vi "RAMP_init_ramp_scan_FPGA.vi"(0 "queue CAMERA":refnum<queue>, 1 "queue piezo":refnum<queue>, 3 "queue DAQ":refnum<queue>, 4 "queue ASI stage":refnum<queue>, 5 "Laser lines array":dbl[][](array[numeric]), 7 "error in":errorcluster, 8 "Illumination source":bool, 9 "Brightfield intensity":dbl, 10 "Display?":bool=TRUE, 12 "Autofocus":bool, 13 "Movie path":path, 14 "Total range (nm)":u32=2000, 15 "z step (nm)":u32=50, 16 "Start acquisition":bool, 17 "Exp time (s)":sgl=0.05 format="%#_3g", 21 "queue FPGA":refnum<queue>, 25 "Measure QPD":bool) -> (20 "Ramp":dbl[](array[numeric]), 23 "Total # z steps":i32, 24 "Ready":bool, 27 "error out":errorcluster)   [LabVIEW 2015]
uses:
  CONTROLS/Q_MCL_piezo_element.ctl
  CONTROLS/Q_camera_element.ctl
  CONTROLS/Q_ASI_stage_element.ctl
  CONTROLS/Q_DAQ_element.ctl
  CONTROLS/Q_FPGA_element.ctl
  GLOBAL/Global_ASI_stage.vi
  GLOBAL/Global_MCL_piezo.vi
  GLOBAL/Global_DAQ.vi
  GLOBAL/Global_CAMERA.vi
  GLOBAL/Global_FPGA.vi
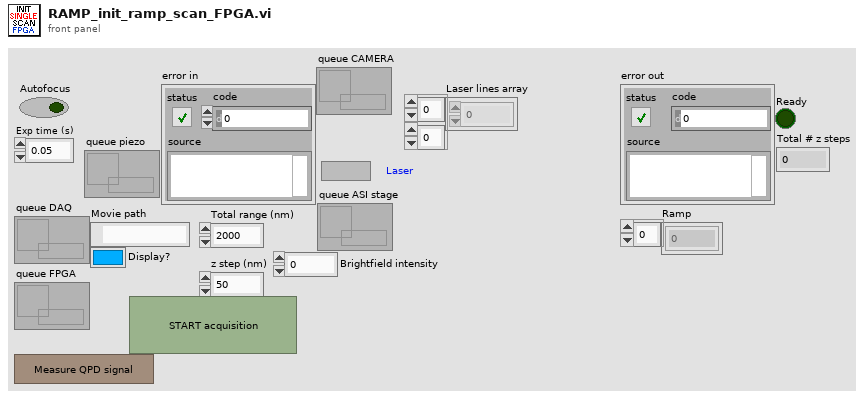
[diagram p1: front panel]
types:
  T1 = typedef "Q_DAQ_element.ctl" = cluster{"variant":variant, "Instruction":enum16{"DAQ_idle", "DAQ_initialize", "DAQ_error", "DAQ_security_stop", "DAQ_init_single_scan", "DAQ_single_scan", "DAQ_init_merFISH", "DAQ_scan_merFISH", "DAQ_photobleaching_merFISH", "DAQ_close_merFISH", "DAQ_stop"}}
  T2 = typedef "Q_camera_element.ctl" = cluster{"variant":variant, "Instruction":enum16{"CAMERA_idle", "CAMERA_initialize", "CAMERA_error", "CAMERA_security_stop", "CAMERA_not_acquiring", "CAMERA_acquiring", "CAMERA_start_acquiring", "CAMERA_stop_acquiring", "CAMERA_change_exposure", "CAMERA_define_ROI", "CAMERA_cooler", "CAMERA_acquire_movie", "CAMERA_init_scan", "CAMERA_check_image_scan", "CAMERA_close_scan", "CAMERA_init_merFISH", "CAMERA_start_acquiring_merFISH", "CAMERA_close_scan_merFISH", "CAMERA_close_merFISH", "CAMERA_STOP"}}
  T3 = cluster{"N laser lines":i32, "N Z positions":i32, "Laser lines":i32[], "Laser power":sgl[], "Measure QPD":bool}
  T4 = typedef "Q_FPGA_element.ctl" = cluster{"variant":variant, "Instruction":enum16{"FPGA_idle", "FPGA_initialize", "FPGA_error", "FPGA_security_stop", "FPGA_laser", "FPGA_start_stop_measure_QPD", "FPGA_measure_QPD", "FPGA_measure_QPD_noise", "FPGA_stop_measure_QPD", "FPGA_init_autofocus", "FPGA_init_single_scan", "FPGA_stop_single_scan", "FPGA_init_merFISH", "FPGA_measure_QPD_merFISH", "FPGA_init_scan_merFISH", "FPGA_scan_merFISH", "FPGA_close_merFISH", "FPGA_stop"}}
  T5 = cluster{"Frames":i32, "Movie path":path, "Start acquisition":bool, "Display?":bool}
  T6 = typedef "Q_MCL_piezo_element.ctl" = cluster{"variant":variant, "Instruction":enum16{"Piezo_idle", "Piezo_initialize", "Piezo_error", "Piezo_security_stop", "Piezo_read_z", "Piezo_move_z", "Piezo_keyboard_move", "Piezo_close_autofocus_calibration_ramp", "Piezo_change_init_state", "Piezo_init_autofocus", "Piezo_init_autofocus_merFISH_TL", "Piezo_autofocus", "Piezo_autofocus_merFISH_TL", "Piezo_stop_autofocus", "Piezo_stop_autofocus_merFISH_TL", "Piezo_autofocus_lost", "Piezo_resume_autofocus_merFISH_TL", "Piezo_check_z_position_merFISH_TL", "Piezo_init_ramp", "Piezo_move_z_ramp", "Piezo_close_ramp", "Piezo_close_merFISH", "Piezo_stop"}}
  T7 = cluster{"Illumination source":bool, "Laser lines array":dbl[][], "Exp time (s)":sgl}
  T8 = typedef "Q_ASI_stage_element.ctl" = cluster{"variant":variant, "Instruction":enum16{"ASI_idle", "ASI_initialize", "ASI_error", "ASI_security_stop", "ASI_read_XYZ", "ASI_up", "ASI_down", "ASI_left", "ASI_right", "ASI_save_XY", "ASI_move_to_XY", "ASI_brightfield", "ASI_init_scan", "ASI_init_merFISH", "ASI_move_to_XY_merFISH", "ASI_move_to_Z_merFISH", "ASI_init_autofocus_search_merFISH", "ASI_close_autofocus_search_merFISH", "ASI_adjust_piezo_autofocus_merFISH", "ASI_set_piezo_autofocus_to_reference_position_merFISH_TL", "ASI_close_merFISH", "ASI_stop"}}
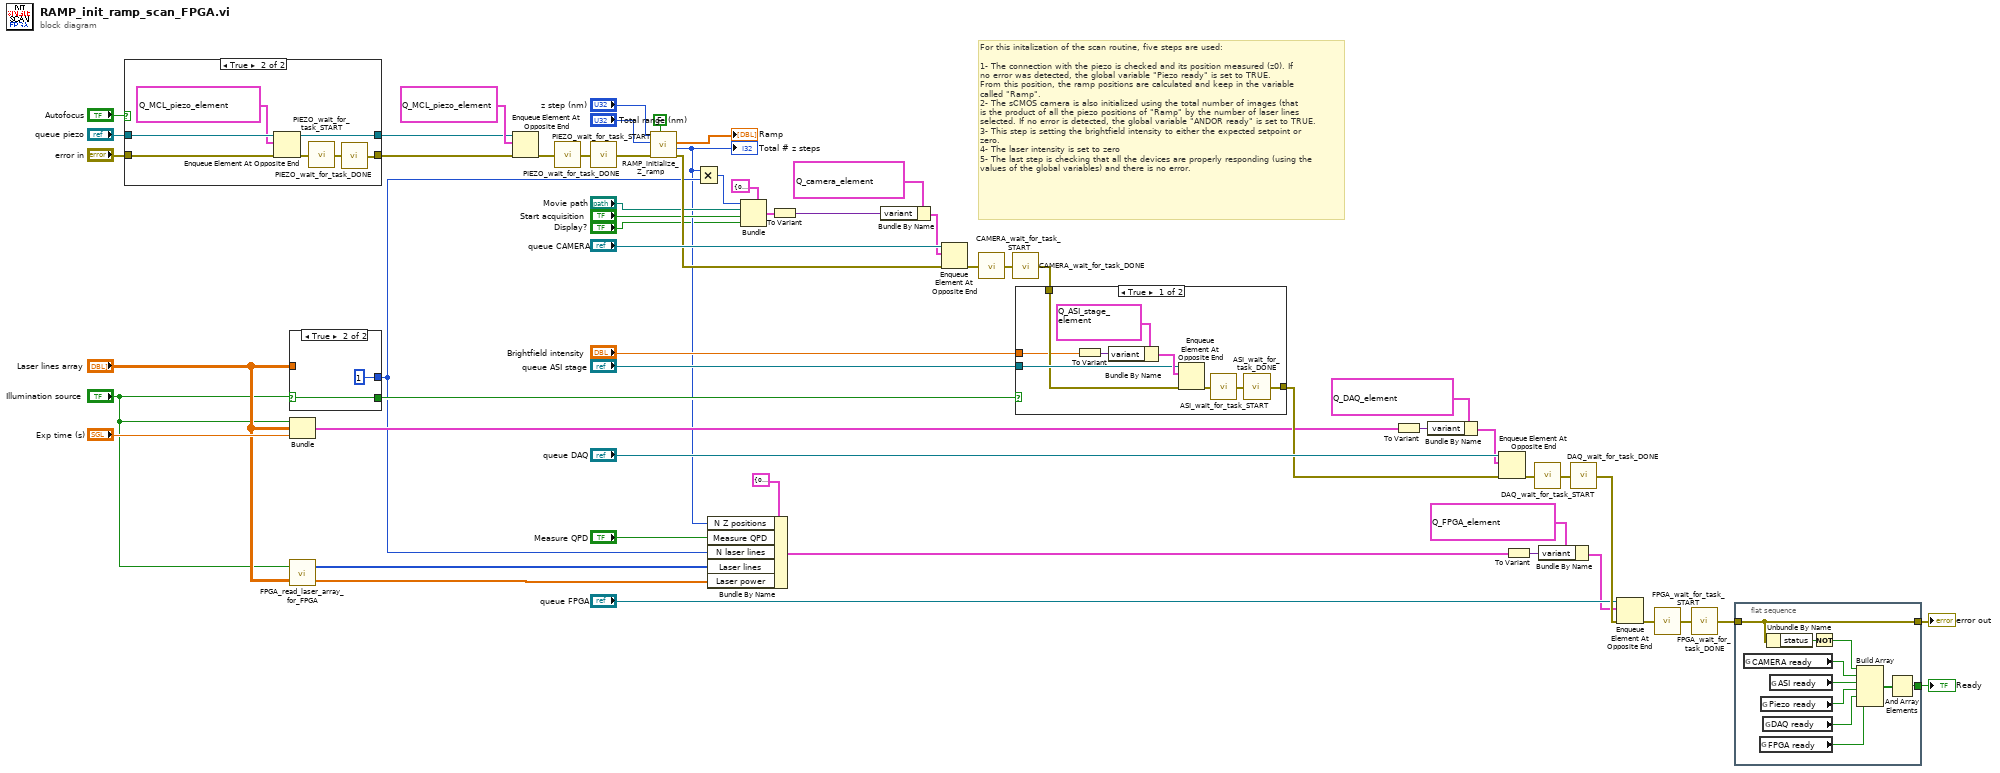
[diagram p0: block diagram]
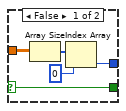
[diagram p2: hidden frame]
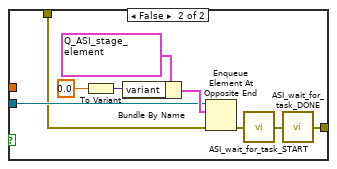
[diagram p4: hidden frame]
diagram:
  # "For this initalization of the scan routine, five steps are used:\n\n1- The connection with the piezo is checked and its position measured (z0). If\nno error was detected, the global variable \"Piezo ready\" is set to TRUE.\nFrom this position, the ramp positions are calculated and keep in the variable \ncalled \"Ramp\".\n2- The sCMOS camera is also initialized using the total number of images (that\nis the product of all the piezo positions of \"Ramp\" by the number of laser lines\nselected. If no error is detected, the global variable \"ANDOR ready\" is set to TRUE.\n3- This step is setting the brightfield intensity to either the expected setpoint or\nzero.\n4- The laser intensity is set to zero\n5- The last step is checking that all the devices are properly responding (using the\nvalues of the global variables) and there is no error."
  n1 = case shown="True" "Autofocus" {
    tunnel: "queue piezo" -> [w59 w67]
    tunnel: [w59 w66] -> w33
    tunnel: "error in" -> [w60 w64]
    tunnel: [w60 w61] -> w31
    frame False {
    }
    frame True {
      n2 = Enqueue Element At Opposite End(queue=w67, element=T6 {"variant"=variant, "Instruction"=enum."Piezo_stop_autofocus"}, error in (no error)=w64) -> (queue out=w66:refnum<queue>, error out=w63:errorcluster)  [unwired: 1 in, 1 out]
      n3 = call "PIEZO_wait_for_task_START.vi"("error in"=w63) -> ("error out"=w62:errorcluster)
      n4 = call "PIEZO_wait_for_task_DONE.vi"("error in"=w62) -> ("error out"=w61:errorcluster)
    }
  }
  n5 = case shown="True" "Illumination source" {
    selector: "Illumination source" -> [w68 w73]
    tunnel: "Laser lines array" -> [w72 _]
    tunnel: [w71 1] -> w21
    tunnel: [w68 w73] -> w28
    frame False {
      n6 = Array Size(array=w72) -> (size(s)=w70:i32[])
      n7 = Index Array(array=w70, index=0) -> (element=w71:i32)
    }
    frame True {
    }
  }
  n8 = Bundle("Illumination source"="Illumination source", "Laser lines array"="Laser lines array", "Exp time (s)"="Exp time (s)") -> (w25:T7)  [unwired: 1 in]
  n9 = call "FPGA_read_laser_array_for_FPGA.vi"("Laser lines array"="Laser lines array", "Illumination source"="Illumination source") -> ("Laser power"=w13:sgl[], "Laser lines"=w14:i32[])
  n10 = Enqueue Element At Opposite End(queue=w33, element=T6 {"variant"=variant, "Instruction"=enum."Piezo_init_ramp"}, error in (no error)=w31) -> (error out=w58:errorcluster)  [unwired: 1 in, 2 out]
  n11 = call "PIEZO_wait_for_task_START.vi"("error in"=w58) -> ("error out"=w57:errorcluster)
  n12 = call "PIEZO_wait_for_task_DONE.vi"("error in"=w57) -> ("error out"=w55:errorcluster)
  n13 = call "RAMP_initialize_Z_ramp.vi"("Symmetric"=FALSE, "error in"=w55, "Total range (nm)"="Total range (nm)", "dZ (nm)"="z step (nm)") -> ("error out"=w51:errorcluster, "Total # steps"=w3:i32, "Ramp"=→"Ramp":dbl[])  [unwired: 1 in, 1 out]
  "Total # z steps" <- w3
  n14 = Multiply(x=w3, y=w21) -> (x*y=w30:i32)
  n15 = Bundle By Name(cluster=T3 {"N laser lines"=0, "N Z positions"=0, "Laser lines"=[0, 0, 0, 0, 0], "Laser power"=[0.0, 0.0, 0.0, 0.0, 0.0], "Measure QPD"=FALSE} ("output cluster"), "N Z positions"=w3, "Measure QPD"="Measure QPD", "N laser lines"=w21, "Laser lines"=w14, "Laser power"=w13) -> (w20:T3)
  n16 = Bundle(cluster=T5 {"Frames"=0, "Movie path"=path "", "Start acquisition"=FALSE, "Display?"=TRUE} ("output cluster"), "Frames"=w30, "Movie path"="Movie path", "Start acquisition"="Start acquisition", "Display?"="Display?") -> (w49:T5)
  n17 = To Variant(anything=w49) -> (Variant=w53:variant)
  n18 = Bundle By Name(cluster=T2 {"variant"=variant, "Instruction"=enum."CAMERA_init_scan"} ("element"), "variant"=w53) -> (w8:T2)
  n19 = Enqueue Element At Opposite End(queue="queue CAMERA", element=w8, error in (no error)=w51) -> (error out=w48:errorcluster)  [unwired: 1 in, 2 out]
  n20 = call "CAMERA_wait_for_task_START.vi"("error in"=w48) -> ("error out"=w47:errorcluster)
  n21 = call "CAMERA_wait_for_task_DONE.vi"("error in"=w47) -> ("error out"=w46:errorcluster)
  n22 = case shown="True" w28 {
    tunnel: w46 -> [w79 w88]
    tunnel: "Brightfield intensity" -> [w75 _]
    tunnel: "queue ASI stage" -> [w80 w89]
    tunnel: [w76 w85] -> w39
    frame True {
      n23 = To Variant(anything=w75) -> (Variant=w82:variant)
      n24 = Bundle By Name(cluster=T8 {"variant"=variant, "Instruction"=enum."ASI_init_scan"} ("Q_ASI_stage"), "variant"=w82) -> (w81:T8)
      n25 = Enqueue Element At Opposite End(queue=w80, element=w81, error in (no error)=w79) -> (error out=w78:errorcluster)  [unwired: 1 in, 2 out]
      n26 = call "ASI_wait_for_task_START.vi"("error in"=w78) -> ("error out"=w77:errorcluster)
      n27 = call "ASI_wait_for_task_DONE.vi"("error in"=w77) -> ("error out"=w76:errorcluster)
    }
    frame False {
      n28 = To Variant(anything=0.0 ("Brightfield intensity")) -> (Variant=w91:variant)
      n29 = Bundle By Name(cluster=T8 {"variant"=variant, "Instruction"=enum."ASI_init_scan"} ("Q_ASI_stage"), "variant"=w91) -> (w90:T8)
      n30 = Enqueue Element At Opposite End(queue=w89, element=w90, error in (no error)=w88) -> (error out=w87:errorcluster)  [unwired: 1 in, 2 out]
      n31 = call "ASI_wait_for_task_START.vi"("error in"=w87) -> ("error out"=w86:errorcluster)
      n32 = call "ASI_wait_for_task_DONE.vi"("error in"=w86) -> ("error out"=w85:errorcluster)
    }
  }
  n33 = To Variant(anything=w25) -> (Variant=w27:variant)
  n34 = Bundle By Name(cluster=T1 {"variant"=variant, "Instruction"=enum."DAQ_init_single_scan"} ("element"), "variant"=w27) -> (w6:T1)
  n35 = Enqueue Element At Opposite End(queue="queue DAQ", element=w6, error in (no error)=w39) -> (error out=w12:errorcluster)  [unwired: 1 in, 2 out]
  n36 = To Variant(anything=w20) -> (Variant=w18:variant)
  n37 = call "DAQ_wait_for_task_START.vi"("error in"=w12) -> ("error out"=w38:errorcluster)
  n38 = Bundle By Name(cluster=T4 {"variant"=variant, "Instruction"=enum."FPGA_init_single_scan"} ("element"), "variant"=w18) -> (w19:T4)
  n39 = call "DAQ_wait_for_task_DONE.vi"("error in"=w38) -> ("error out"=w24:errorcluster)
  n40 = Enqueue Element At Opposite End(queue="queue FPGA", element=w19, error in (no error)=w24) -> (error out=w17:errorcluster)  [unwired: 1 in, 2 out]
  n41 = call "FPGA_wait_for_task_START.vi"("error in"=w17) -> ("error out"=w16:errorcluster)
  n42 = call "FPGA_wait_for_task_DONE.vi"("error in"=w16) -> ("error out"=w15:errorcluster)
  n43 = flat-sequence {
    tunnel: [w102] -> w36
    tunnel: w15 -> [w95]
    tunnel: [w95] -> w37
    frame #0 {
      n44 = global read "Global_CAMERA.vi" "CAMERA ready"() -> (w99:bool)
      n45 = global read "Global_FPGA.vi" "FPGA ready"() -> (w93:bool)
      n46 = global read "Global_MCL_piezo.vi" "Piezo ready"() -> (w100:bool)
      n47 = global read "Global_DAQ.vi" "DAQ ready"() -> (w94:bool)
      n48 = Unbundle By Name(w95) -> ("status"=w97:bool)
      n49 = global read "Global_ASI_stage.vi" "ASI ready"() -> (w101:bool)
      n50 = Not(x=w97) -> (.not. x?=w96:bool)
      n51 = Build Array(w96, w99, w101, w100, w94, w93) -> (w98:bool[])
      n52 = And Array Elements(Boolean array=w98) -> (logical AND=w102:bool)
    }
  }
  "error out" <- w37
  "Ready" <- w36
